vi "DimostratoreCalibrazioni.vi"() -> ()   [LabVIEW 2019]
uses:
  TypeDef/SlugExpiration.ctl
  ByteGSAPIBase.lvclass
  TypeDef/CalibrationStates.ctl
  FetchCalibration/Converted_Slug_Cluster.ctl
  Instruments/Instruments.ctl
  CalibrationMeasurements/BodyCalibrazioneMisure.ctl
  aa47c742-c095-4670-bf1f-6b28e4309cef.vi
  <vilib>/numeric/Random Number (Range) I64.vi
  <vilib>/Array/Sort 2D Array - Pop Stack.vi
  <vilib>/Array/Sort 2D Array - Push Stack.vi
  <vilib>/numeric/sub_Random U32.vi
panel:
  out "Stato":string
  out "Misurazione n.":string
  in  "Cancel":bool
  in  "Approvation":bool
  out "Tot Misurazioni":i32
  in  "Avanti":bool
  in  "Repeat":bool
  out "Esito":string
  out "Valore misurato":dbl
  out "Valore di riferimento":dbl
  out "Waveform Chart":i64(graph)
  in  "Start Calibration":bool
  in  "Next":bool
  in  "Previus":bool
  out "Calibrazioni n.":string
  in  "Filtro":enum16{"All", "Expired", "Not Expired"}(ring)
  in  "Slug list":T1[](array[typedef])
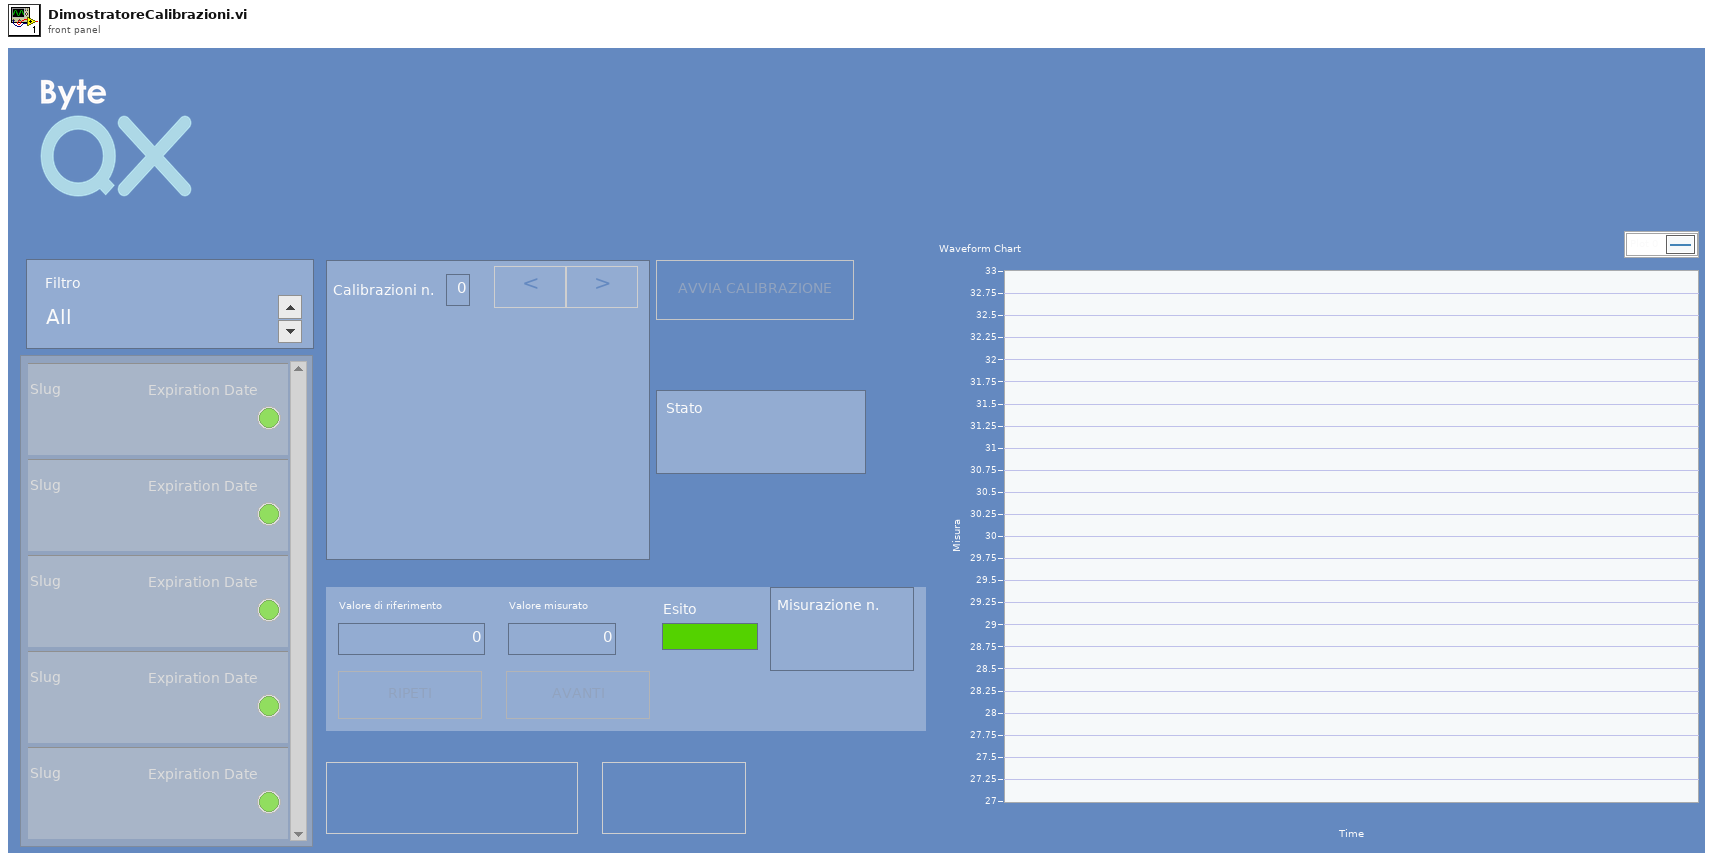
[diagram p1: front panel]
types:
  T1 = typedef "SlugExpiration.ctl" = cluster{"Slug":string, "Expiration Date":string, "Color Box":u32, "Active":bool, "Expired?":bool, "Id":i32}
  T2 = typedef "CalibrationStates.ctl" = enum16{"Init", "Idle", "GetInstruments", "Fetch", "GetCalibrations", "CheckTotalMisurations", "StartCalibration", "ManageCalibration", "AllowApprove", "Approve"}
  T3 = typedef "ByteGSWebAPI.lvlib/ByteGSAPIBase.lvclass/BodyCalibrazioneMisure.ctl" = cluster{"controls":cluster{"id":u16, "descrizione":string, "numero_misure_necessarie":u16, "riferimento_obiettivo":dbl, "mpe_max":dbl, "mpe_min":dbl, "deviazione_standard":dbl, "incertezza":dbl, "numero_misure_effettuate":u32, "temperatura_c":dbl, "umidita":dbl, "strumento_riferimento":cluster{"id":u16, "nome":string}[]}[]}
  T4 = typedef "Instruments.ctl" = cluster{"id":i32, "slug":string, "stabilimento":cluster{"id":dbl}, "categoria":cluster{"id":dbl}, "tipologia_di_visualizzazione":cluster{"id":dbl}, "stato":cluster{"id":dbl}, "descrizione":string, "costruttore":string, "matricola":string, "data_registrazione":string, "intervallo_di_taratura_mesi":dbl, "reparto":string, "campo_misura":string, "risoluzione":dbl, "responsabile_strumento":string, "classe_di_precisione":string, "classificazione":string, "appunti":string, "manuale":string, "foto":string, "riferimento":bool, "qr_hashcode":string, "costo_euro":dbl}
  T5 = typedef "ByteGSWebAPI.lvlib/ByteGSAPIBase.lvclass/Converted_Slug_Cluster.ctl" = cluster{"id":u32, "instrument":string, "name":string, "date":timestamp}
  T6 = cluster{"Esito":refnum<vi>, "Avanti":refnum<vi>, "Repeat":refnum<vi>, "Slug list":refnum<vi>, "Start Calibration":refnum<vi>, "Avanti":refnum<vi>, "Cancel":refnum<vi>, "Approvation":refnum<vi>}
  T7 = cluster{"ByteGSAPIBase in":refnum<class "ByteGSAPIBase.lvclass">, "Instruments_Slug":string[], "All_Instruments_Cals":T5[], "All_Instruments":T4[], "Slug list All":T1[], "Calibrations":T3, "Selected Slug":i32, "Misurazioni":string, "Misurazioni index":i32, "Next State":T2, "Waveform Chart":refnum<vi>, "New Val":dbl, "Id Failed":u32, "Failed?":bool, "Cal Index":i32, "Misurazioni n":string, "Stato":string, "Esito":string, "Misure effettuate":i32}
  T8 = cluster{"id":u16, "descrizione":string, "numero_misure_necessarie":u16, "riferimento_obiettivo":dbl, "mpe_max":dbl, "mpe_min":dbl, "deviazione_standard":dbl, "incertezza":dbl, "numero_misure_effettuate":u32, "temperatura_c":dbl, "umidita":dbl, "strumento_riferimento":cluster{"id":u16, "nome":string}[]}[]
  T9 = cluster{"id":u16, "descrizione":string, "numero_misure_necessarie":u16, "riferimento_obiettivo":dbl, "mpe_max":dbl, "mpe_min":dbl, "deviazione_standard":dbl, "incertezza":dbl, "numero_misure_effettuate":u32, "temperatura_c":dbl, "umidita":dbl, "strumento_riferimento":cluster{"id":u16, "nome":string}[]}
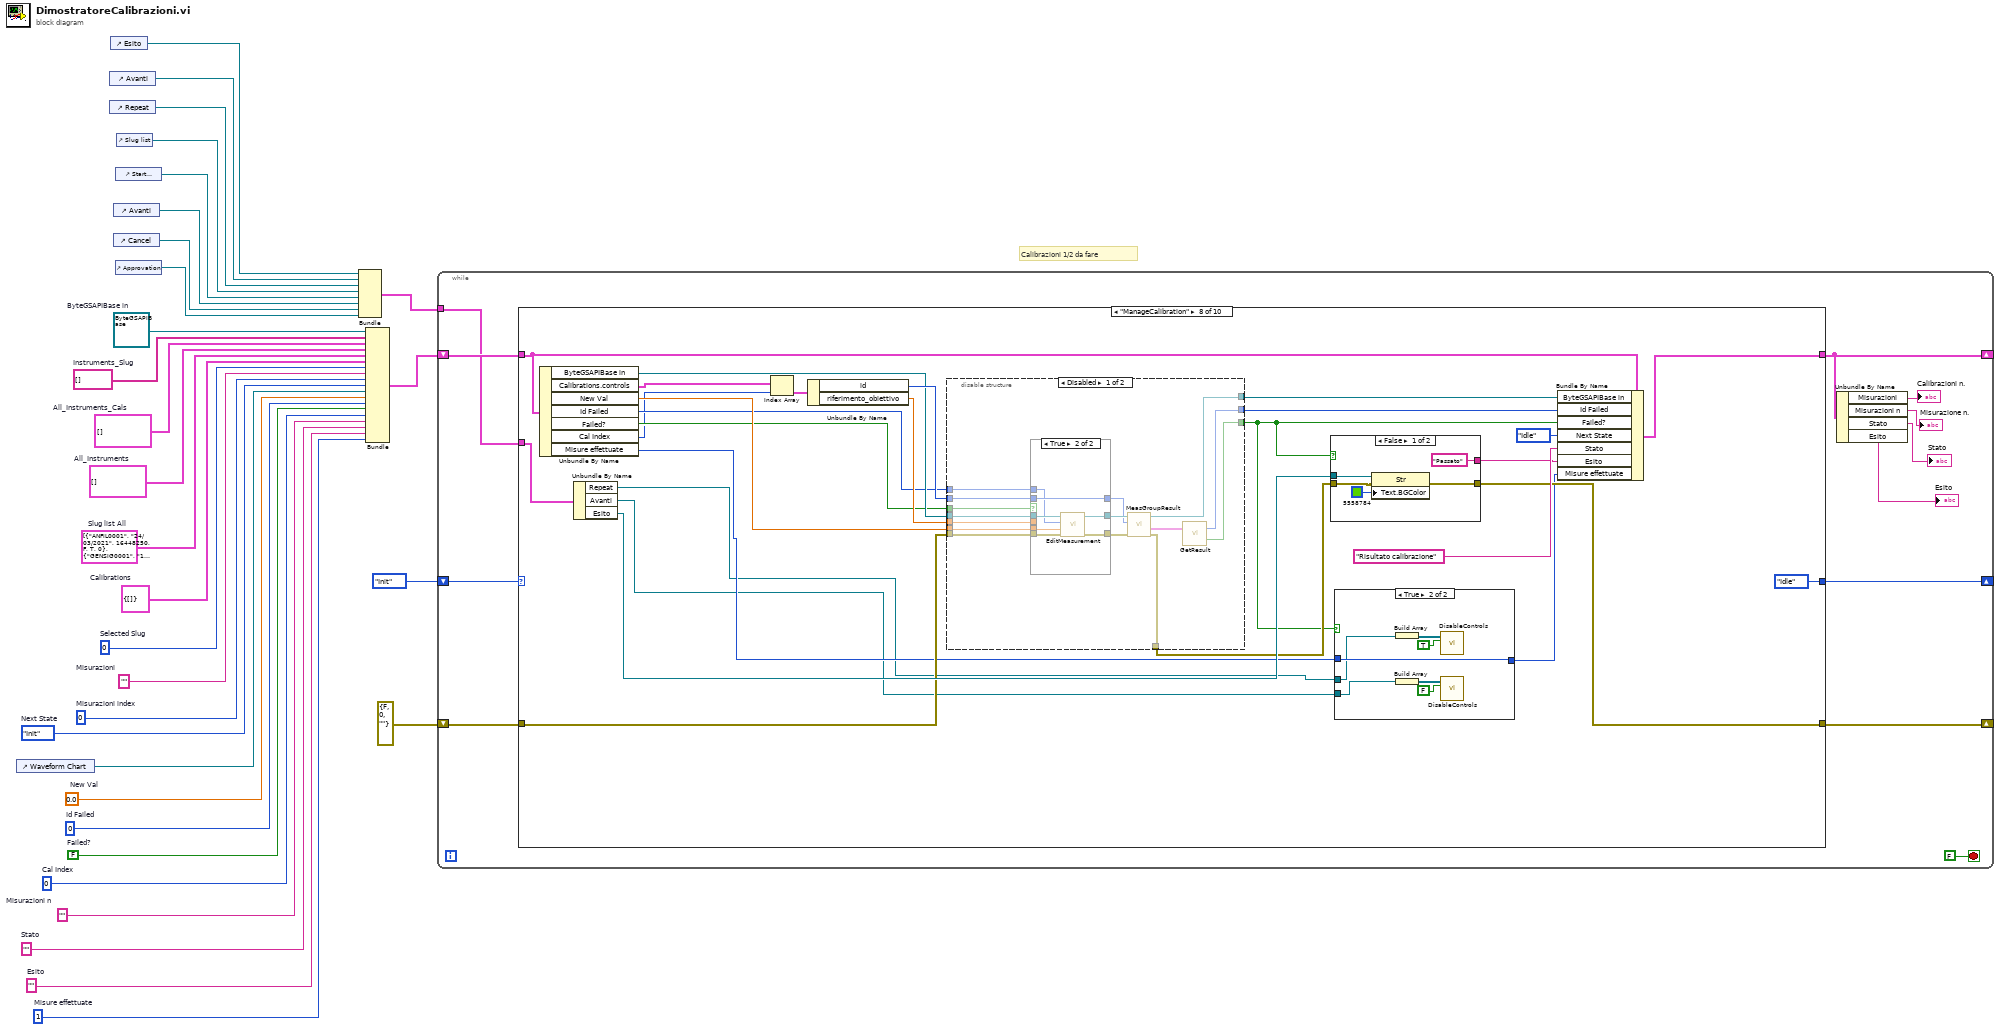
[diagram p0: block diagram]
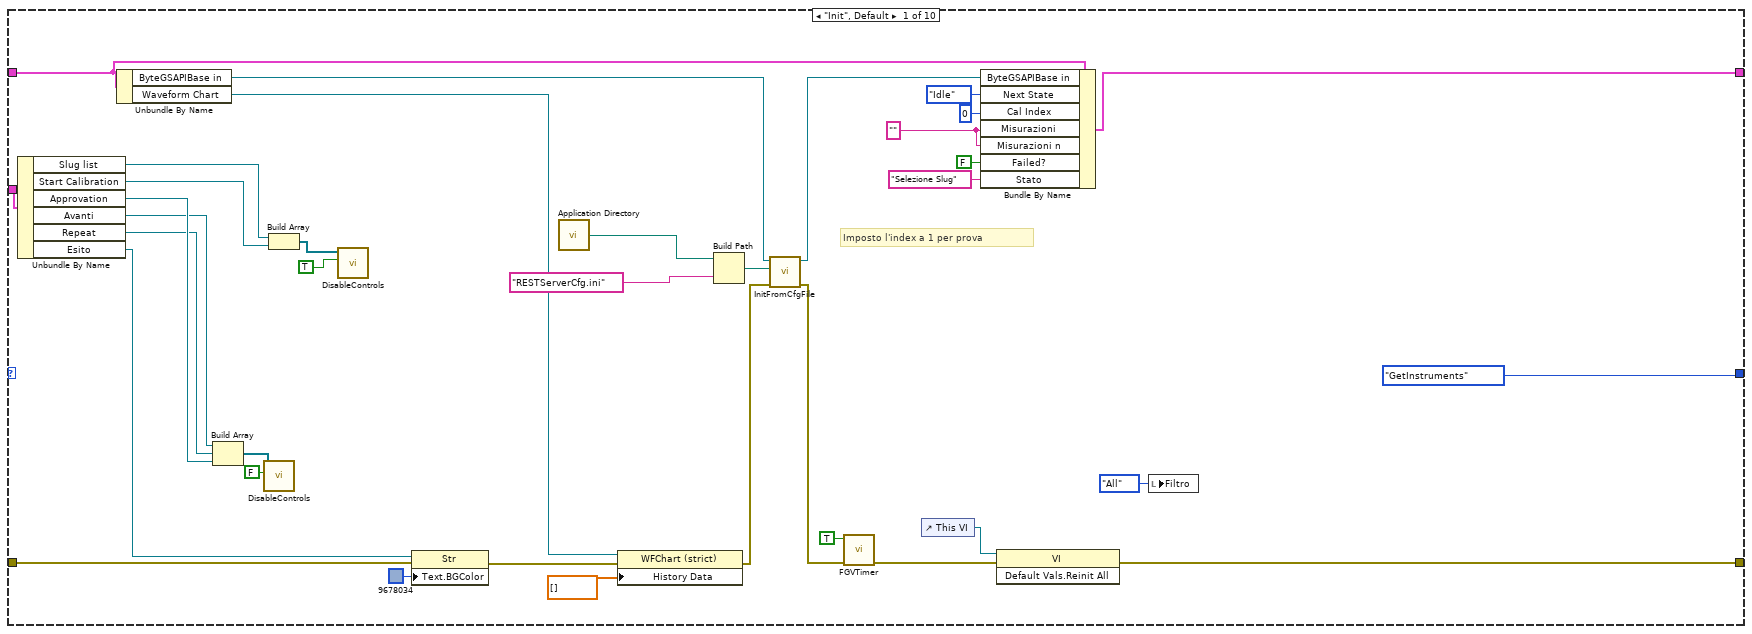
[diagram p2: hidden frame]
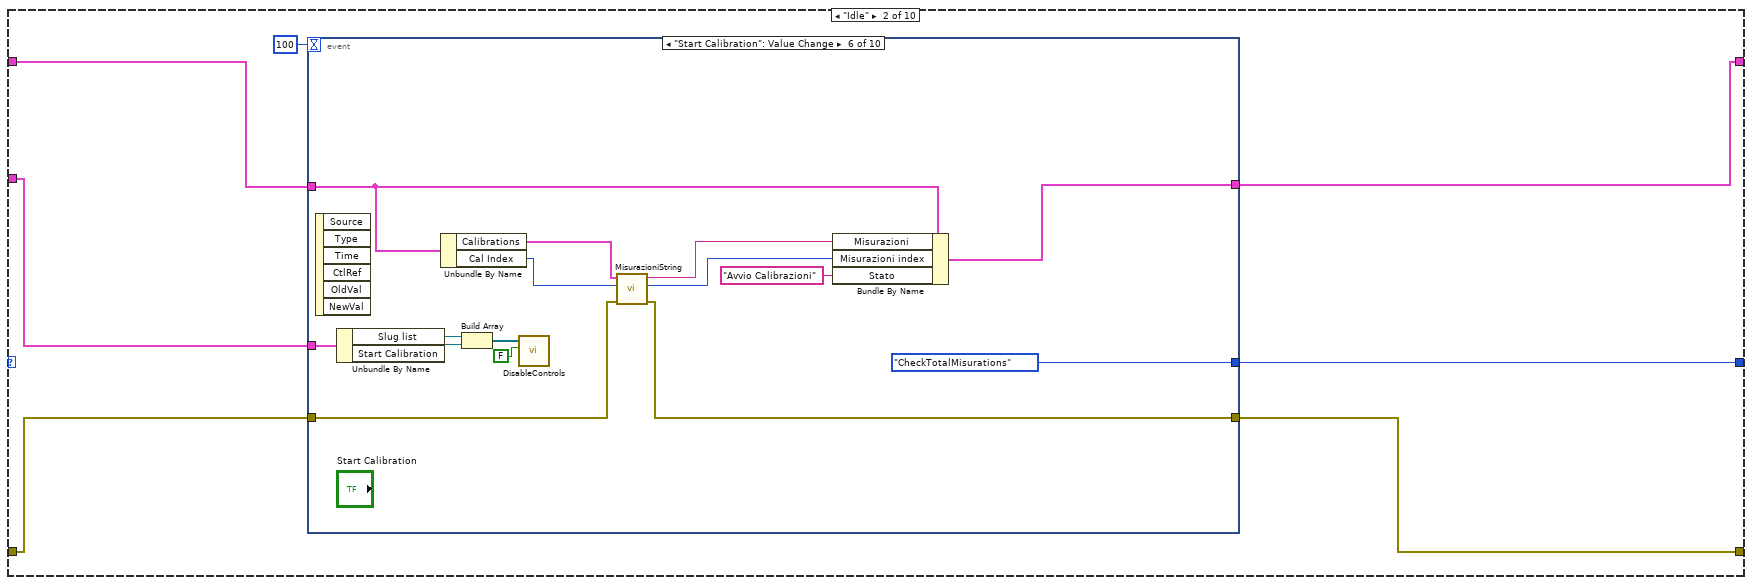
[diagram p3: hidden frame]
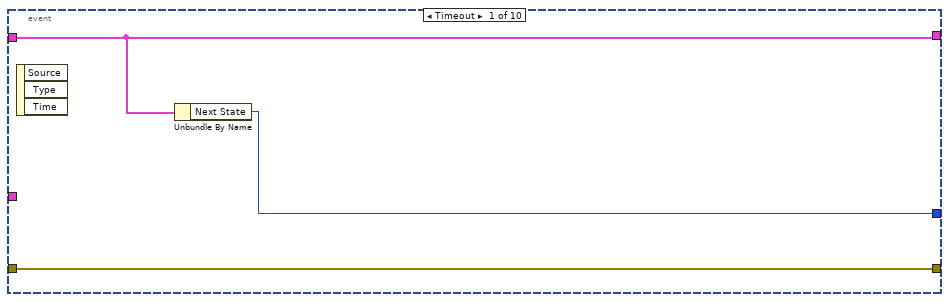
[diagram p4: hidden frame]
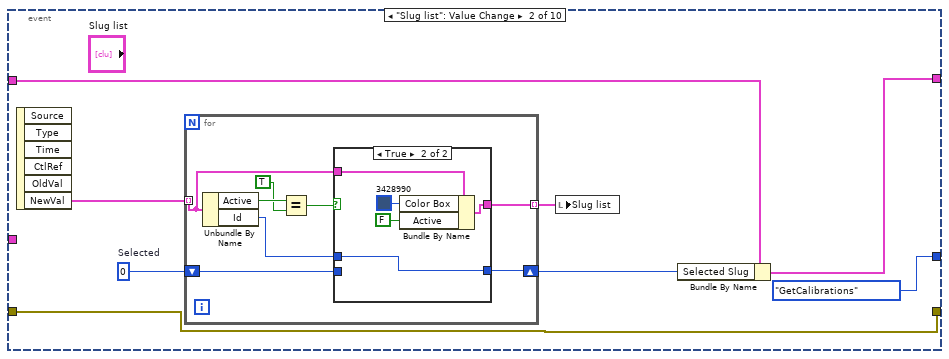
[diagram p5: hidden frame]
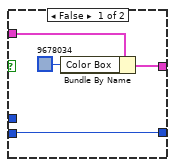
[diagram p6: hidden frame]
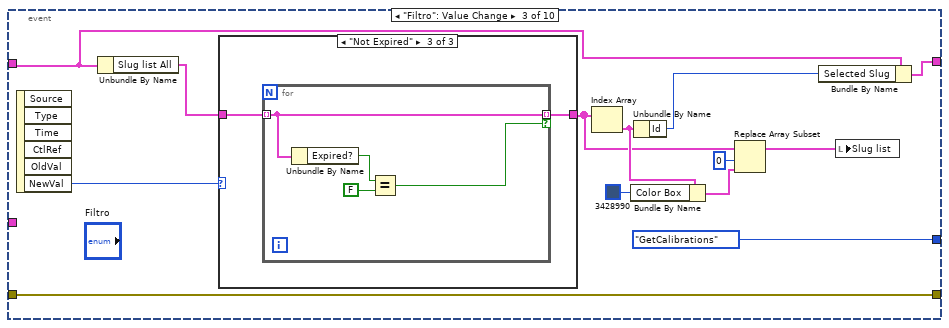
[diagram p7: hidden frame]
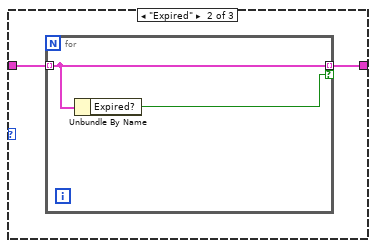
[diagram p9: hidden frame]
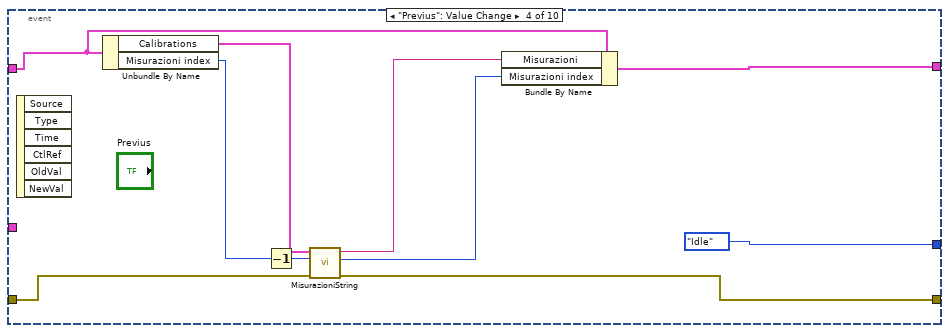
[diagram p10: hidden frame]
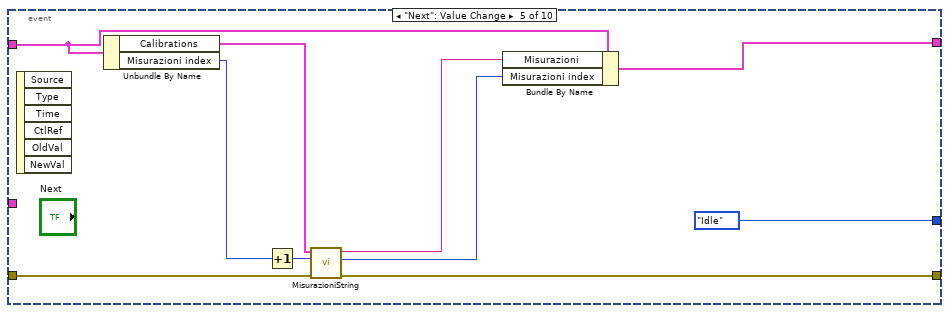
[diagram p11: hidden frame]
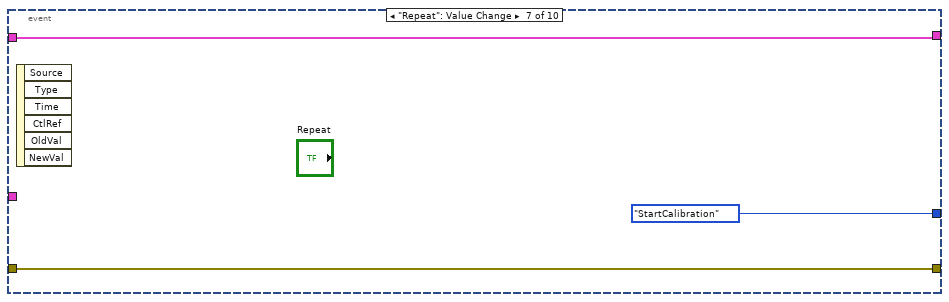
[diagram p12: hidden frame]
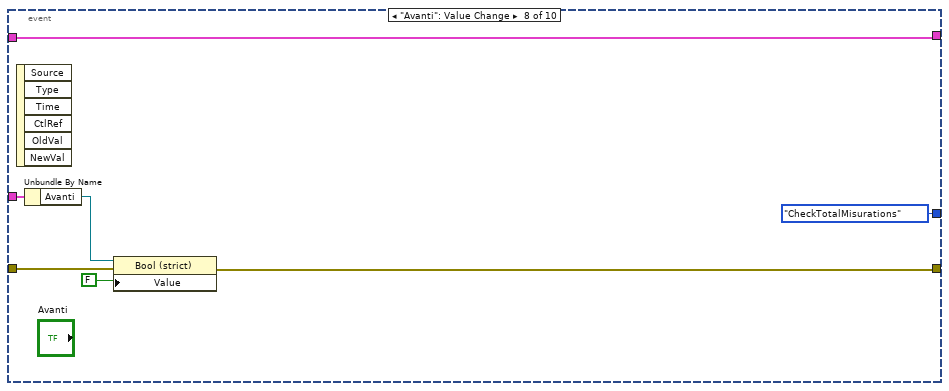
[diagram p13: hidden frame]
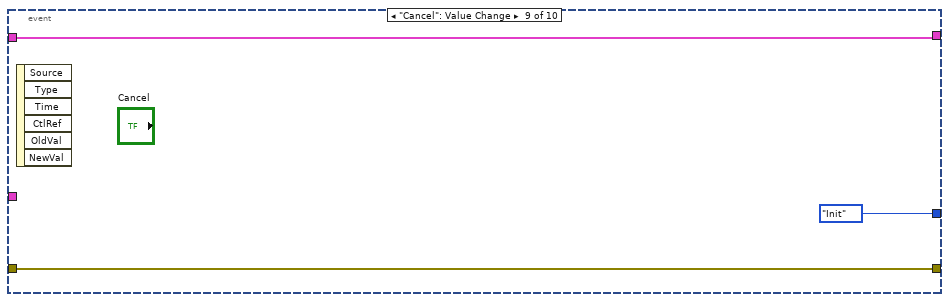
[diagram p14: hidden frame]
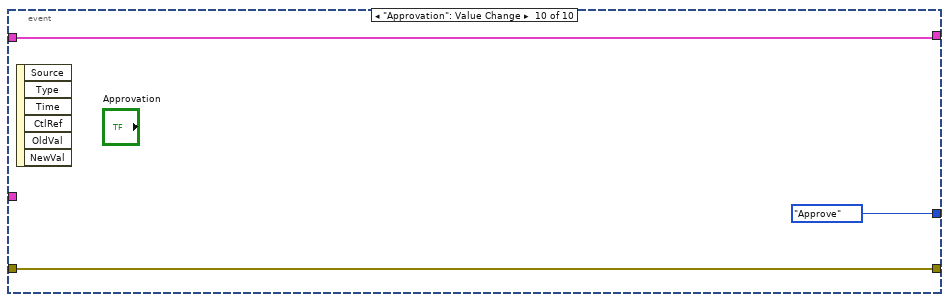
[diagram p15: hidden frame]
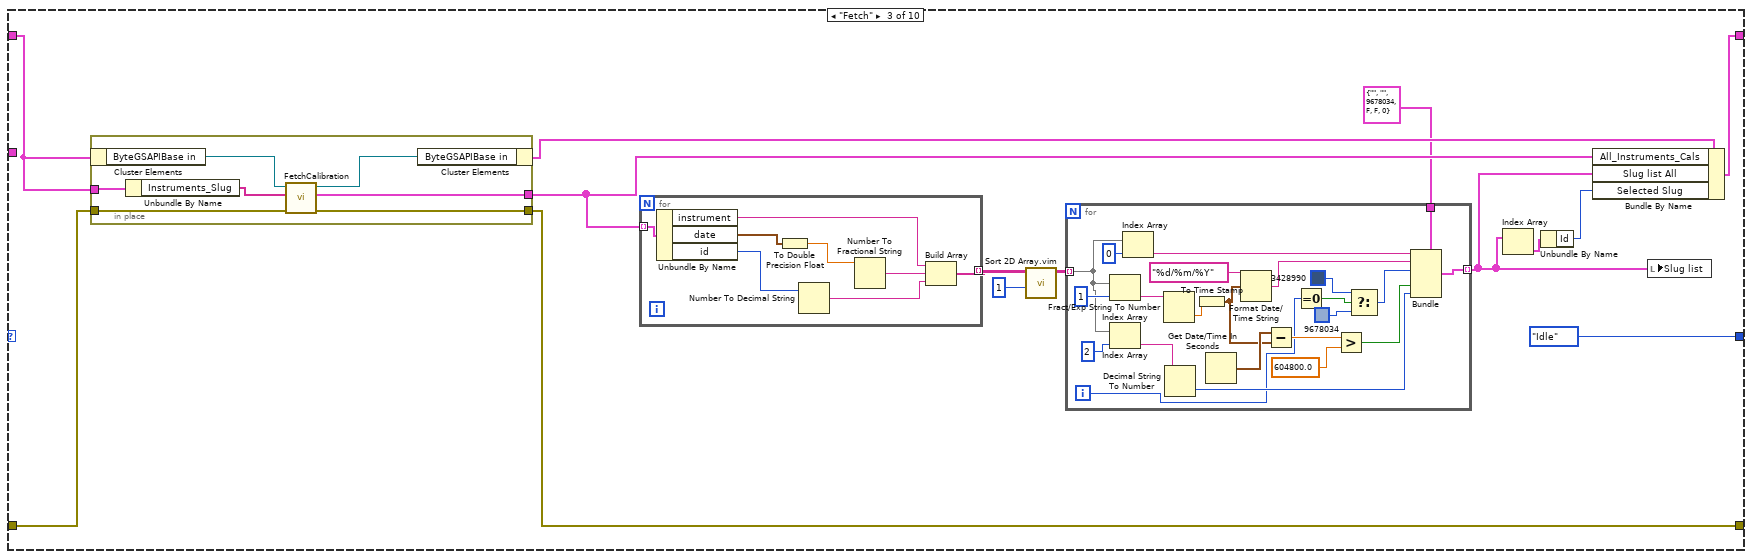
[diagram p16: hidden frame]
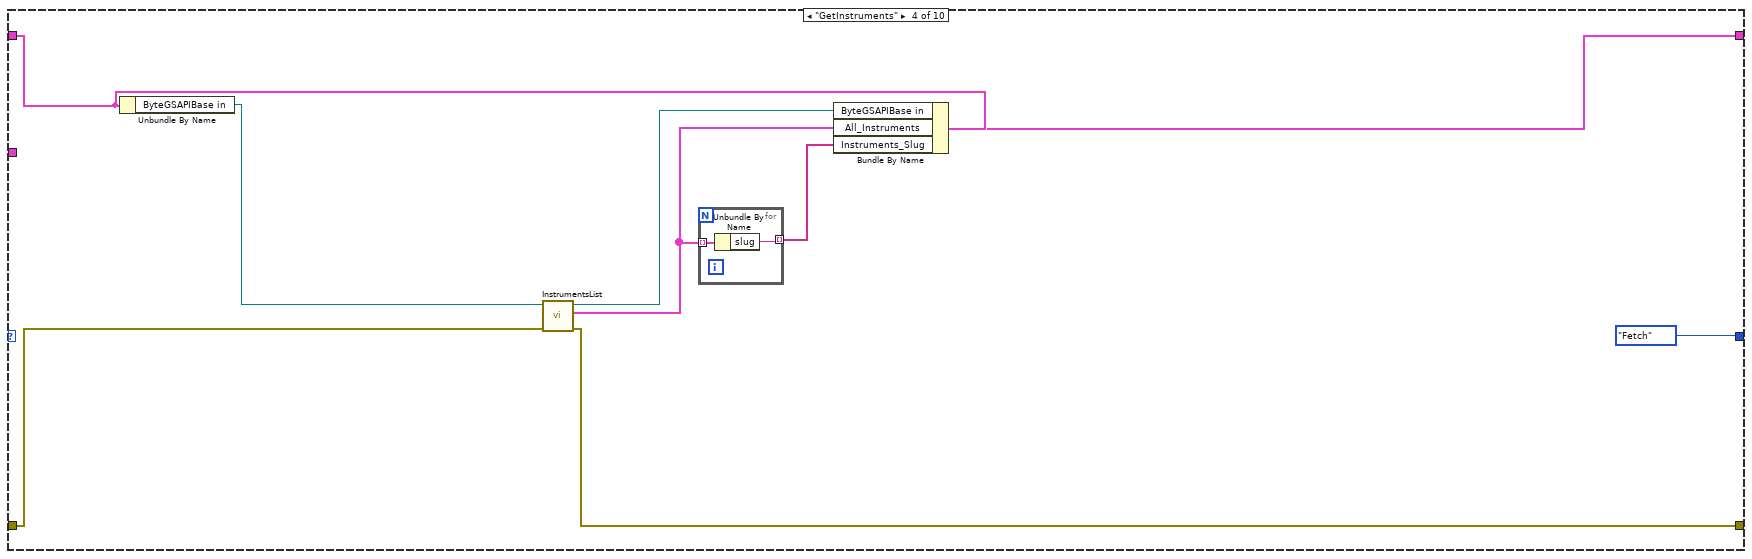
[diagram p17: hidden frame]
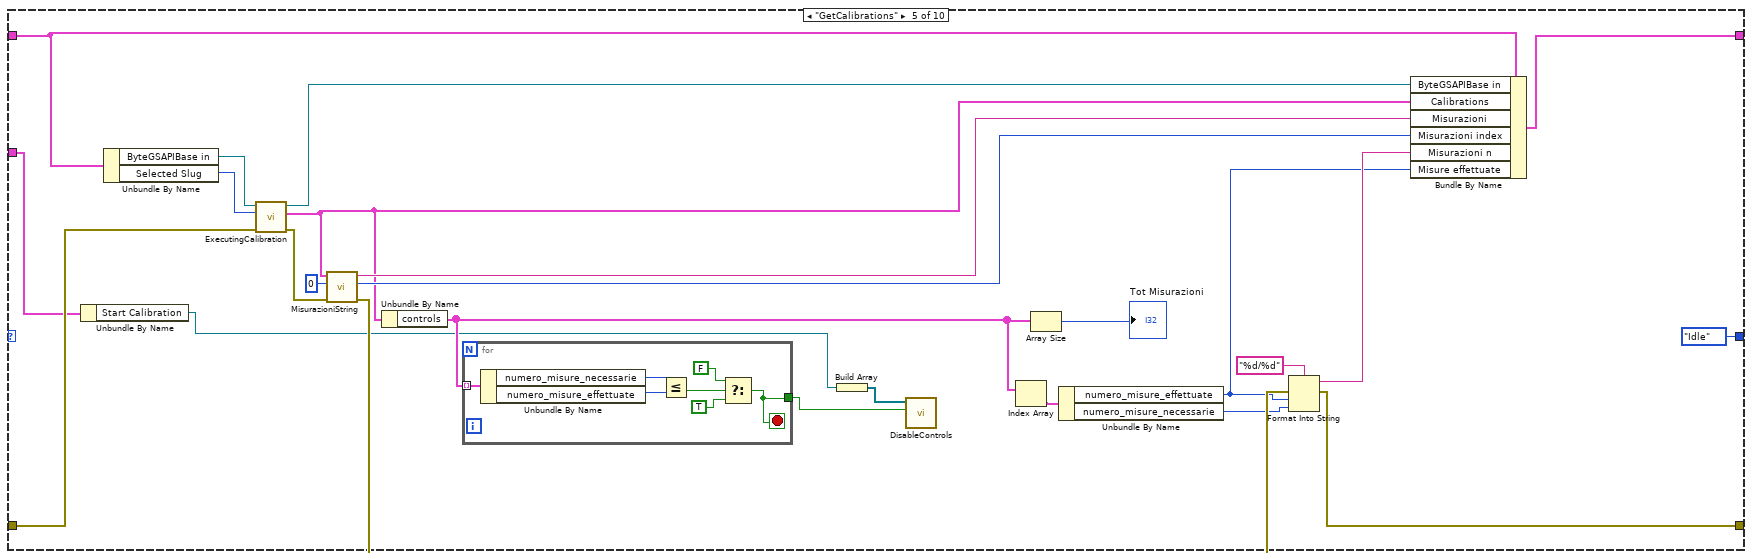
[diagram p18: hidden frame]
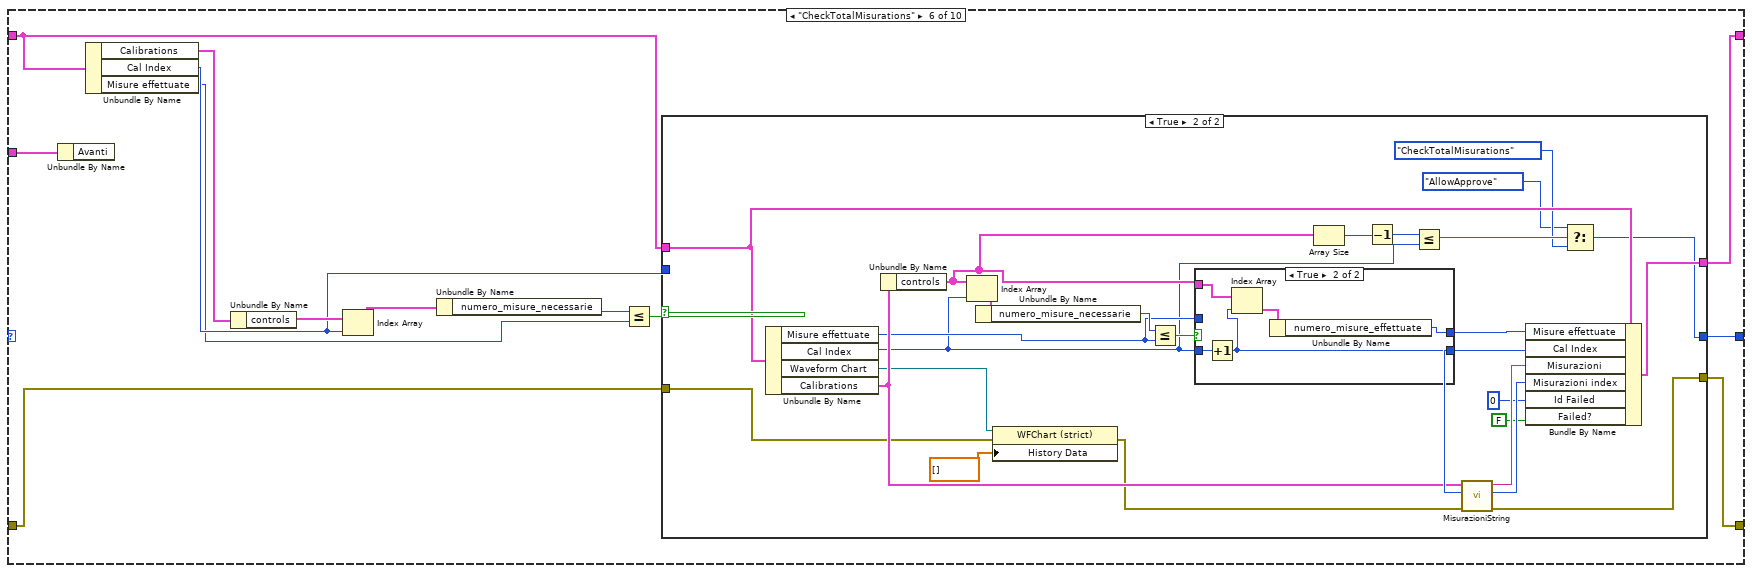
[diagram p19: hidden frame]
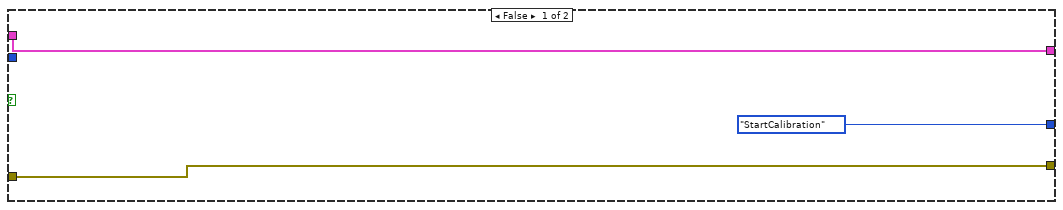
[diagram p20: hidden frame]
diagram:
  w1 = 1  # Misure effettuate
  w3 = ""  # Esito
  w4 = ""  # Stato
  w9 = ""  # Misurazioni n
  w14 = 0  # Cal Index
  w15 = FALSE  # Failed?
  w16 = u32 0  # Id Failed
  w17 = 0.0  # New Val
  w19 = CalibrationStates."Init"  # Next State
  w20 = 0  # Misurazioni index
  w21 = ""  # Misurazioni
  w22 = T1[] [{"Slug"="ANFIL0001", "Expiration Date"="24/03/2021", "Color Box"=16448250, "Active"=FALSE, "Expired?"=TRUE, "Id"=0}, {"Slug"="GENSIG0001", "Expiration Date"="18/05/2021", "Color Box"=16448250, "Active"=FALSE, "Expired?"=TRUE, "Id"=0}, {"Slug"="GENSIG0001", "Expiration Date"="15/09/2021", "Color Box"=16448250, "Active"=FALSE, "Expired?"=TRUE, "Id"=0}, {"Slug"="DIN0001", "Expiration Date"="11/10/2021", "Color Box"=13816530, "Active"=FALSE, "Expired?"=TRUE, "Id"=0}, {"Slug"="DMM0002", "Expiration Date"="20/10/2021", "Color Box"=16448250, "Active"=FALSE, "Expired?"=TRUE, "Id"=0}, {"Slug"="COMP0001", "Expiration Date"="01/12/2021", "Color Box"=16448250, "Active"=FALSE, "Expired?"=TRUE, "Id"=0}, {"Slug"="TORS0002", "Expiration Date"="06/12/2021", "Color Box"=16448250, "Active"=FALSE, "Expired?"=TRUE, "Id"=0}, {"Slug"="CDIND0001", "Expiration Date"="04/03/2022", "Color Box"=16448250, "Active"=FALSE, "Expired?"=TRUE, "Id"=0}, {"Slug"="CALI0004", "Expiration Date"="11/03/2022", "Color Box"=16448250, "Active"=FALSE, "Expired?"=TRUE, "Id"=0}, {"Slug"="CALI0001", "Expiration Date"="10/05/2022", "Color Box"=16448250, "Active"=FALSE, "Expired?"=TRUE, "Id"=0}, {"Slug"="CALI0012", "Expiration Date"="10/05/2022", "Color Box"=16448250, "Active"=FALSE, "Expired?"=TRUE, "Id"=0}, {"Slug"="CALI0011", "Expiration Date"="11/05/2022", "Color Box"=16448250, "Active"=FALSE, "Expired?"=TRUE, "Id"=0}, {"Slug"="CALI0014", "Expiration Date"="04/07/2022", "Color Box"=16448250, "Active"=FALSE, "Expired?"=TRUE, "Id"=0}, {"Slug"="CDIND0001", "Expiration Date"="15/07/2022", "Color Box"=16448250, "Active"=FALSE, "Expired?"=TRUE, "Id"=0}, {"Slug"="CALI0024", "Expiration Date"="11/07/2023", "Color Box"=16448250, "Active"=FALSE, "Expired?"=TRUE, "Id"=0}, {"Slug"="CALI0017", "Expiration Date"="19/09/2023", "Color Box"=16448250, "Active"=FALSE, "Expired?"=TRUE, "Id"=0}, {"Slug"="CALI0020", "Expiration Date"="02/11/2023", "Color Box"=16448250, "Active"=FALSE, "Expired?"=TRUE, "Id"=0}, {"Slug"="CALI0017", "Expiration Date"="03/11/2023", "Color Box"=16448250, "Active"=FALSE, "Expired?"=TRUE, "Id"=0}, {"Slug"="CALI0025", "Expiration Date"="11/11/2023", "Color Box"=16448250, "Active"=FALSE, "Expired?"=TRUE, "Id"=0}, {"Slug"="CLBR0001", "Expiration Date"="30/11/2023", "Color Box"=16448250, "Active"=FALSE, "Expired?"=TRUE, "Id"=0}, {"Slug"="CLBR0001", "Expiration Date"="02/01/2024", "Color Box"=16448250, "Active"=FALSE, "Expired?"=TRUE, "Id"=0}, {"Slug"="CLBR0001", "Expiration Date"="02/01/2024", "Color Box"=16448250, "Active"=FALSE, "Expired?"=TRUE, "Id"=0}, {"Slug"="CLBR0003", "Expiration Date"="04/03/2024", "Color Box"=16448250, "Active"=FALSE, "Expired?"=TRUE, "Id"=0}, {"Slug"="MICP0001", "Expiration Date"="19/03/2024", "Color Box"=16448250, "Active"=FALSE, "Expired?"=TRUE, "Id"=0}, {"Slug"="TERM0002", "Expiration Date"="04/07/2024", "Color Box"=16448250, "Active"=FALSE, "Expired?"=TRUE, "Id"=0}, {"Slug"="ACCEL0008", "Expiration Date"="04/07/2024", "Color Box"=16448250, "Active"=FALSE, "Expired?"=TRUE, "Id"=0}, {"Slug"="ACCEL0008", "Expiration Date"="05/07/2024", "Color Box"=16448250, "Active"=FALSE, "Expired?"=TRUE, "Id"=0}, {"Slug"="ACCEL0008", "Expiration Date"="19/08/2024", "Color Box"=16448250, "Active"=FALSE, "Expired?"=TRUE, "Id"=0}, {"Slug"="TERM0002", "Expiration Date"="15/10/2024", "Color Box"=16448250, "Active"=FALSE, "Expired?"=TRUE, "Id"=0}, {"Slug"="BILA0001", "Expiration Date"="15/10/2024", "Color Box"=16448250, "Active"=FALSE, "Expired?"=TRUE, "Id"=0}, {"Slug"="CLBR0001", "Expiration Date"="15/10/2024", "Color Box"=16448250, "Active"=FALSE, "Expired?"=TRUE, "Id"=0}, {"Slug"="ACCEL0002", "Expiration Date"="15/10/2024", "Color Box"=16448250, "Active"=FALSE, "Expired?"=TRUE, "Id"=0}]  # Slug list All
  w23 = 0  # Selected Slug
  w24 = T3 {"controls"=[]}  # Calibrations
  w25 = T4[] []  # All_Instruments
  w26 = T5[] []  # All_Instruments_Cals
  w27 = string[] []  # Instruments_Slug
  w30 = refnum<class "ByteGSAPIBase.lvclass"> refnum  # ByteGSAPIBase in
  # "Calibrazioni 1/2 da fare"
  n1 = control-ref of="Waveform Chart"() -> (w18:refnum<vi>)
  n2 = control-ref of="Avanti"() -> (w5:refnum<vi>)
  n3 = control-ref of="Repeat"() -> (w6:refnum<vi>)
  n4 = control-ref of="Esito"() -> (w2:refnum<vi>)
  n5 = control-ref of="Avanti"() -> (w10:refnum<vi>)
  n6 = control-ref of="Cancel"() -> (w11:refnum<vi>)
  n7 = control-ref of="Start Calibration"() -> (w8:refnum<vi>)
  n8 = control-ref of="Approvation"() -> (w12:refnum<vi>)
  n9 = control-ref of="Slug list"() -> (w7:refnum<vi>)
  n10 = Bundle("Esito"=w2, "Avanti"=w5, "Repeat"=w6, "Slug list"=w7, "Start Calibration"=w8, "Avanti"=w10, "Cancel"=w11, "Approvation"=w12) -> (w13:T6)  [unwired: 1 in]
  n11 = Bundle("ByteGSAPIBase in"=w30, "Instruments_Slug"=w27, "All_Instruments_Cals"=w26, "All_Instruments"=w25, "Slug list All"=w22, "Calibrations"=w24, "Selected Slug"=w23, "Misurazioni"=w21, "Misurazioni index"=w20, "Next State"=w19, "Waveform Chart"=w18, "New Val"=w17, "Id Failed"=w16, "Failed?"=w15, "Cal Index"=w14, "Misurazioni n"=w9, "Stato"=w4, "Esito"=w3, "Misure effettuate"=w1) -> (w29:T7)  [unwired: 1 in]
  n12 = while {
    shift-right: [w41] -> _
    shift-left: CalibrationStates."Init" -> [w42]
    shift-right: [w37] -> _
    shift-left: w29 -> [w40]
    shift-right: [w38] -> _
    shift-left: errorcluster {"status"=FALSE, "code"=0, "source"=""} ("error in (no error)") -> [w39]
    tunnel: w13 -> [w35]
    stop <- FALSE stop-if-true
    n13 = case shown="\"ManageCalibration\"" w42 {
      tunnel: [CalibrationStates."GetInstruments" w84 CalibrationStates."Idle" CalibrationStates."Fetch" CalibrationStates."Idle" w292 CalibrationStates."Idle" CalibrationStates."Idle" CalibrationStates."Idle" CalibrationStates."Idle"] -> w41
      tunnel: w40 -> [w75 w86 w203 w248 w273 w288 w359 w395 w462 w496]
      tunnel: w39 -> [w45 w83 w202 w250 w274 w290 w343 w381 w465 w495]
      tunnel: [w61 w82 w195 w244 w264 w289 w351 w382 w465 w493] -> w38
      tunnel: [w73 w85 w199 w246 w272 w287 w358 w394 w462 w487] -> w37
      tunnel: w35 -> [w63 w80 _ _ w256 w291 w347 w387 w471 w492]
      frame "Init", Default {
        w59 = "" ("Misurazioni")
        # "Imposto l'index a 1 per prova"
        n14 = Unbundle By Name(w63) -> ("Slug list"=w57:refnum<vi>, "Start Calibration"=w56:refnum<vi>, "Approvation"=w58:refnum<vi>, "Avanti"=w51:refnum<vi>, "Repeat"=w50:refnum<vi>, "Esito"=w44:refnum<vi>)
        n15 = Unbundle By Name(w75) -> ("ByteGSAPIBase in"=w76:refnum<class "ByteGSAPIBase.lvclass">, "Waveform Chart"=w67:refnum<vi>)
        n16 = Build Array(w51, w50, w58) -> (w53:refnum<vi>[])
        n17 = call "DisableControls.vi"("Visible"=FALSE, "Controls"=w53) -> ()  [unwired: 9 in, 1 out]
        n18 = Build Array(w57, w56) -> (w55:refnum<vi>[])
        n19 = call "DisableControls.vi"("Visible"=TRUE, "Controls"=w55) -> ()  [unwired: 9 in, 1 out]
        n20 = property class="Str"(reference=w44, error in=w45, "Text.BGColor"=u32 9678034 ("Text.Text Colors:BG Color")) -> (error out=w46:errorcluster)  [unwired: 1 out]
        n21 = call <vilib>:"Application Directory.vi"() -> ("Application Directory"=w77:path)
        n22 = property class="WFChart (strict)"(reference=w67, error in=w46, "History Data"=dbl[] []) -> (error out=w66:errorcluster)  [unwired: 1 out]
        n23 = Build Path(base path=w77, name or relative path="RESTServerCfg.ini") -> (appended path=w72:path)
        n24 = call-dynamic "InitFromCfgFile.vi"("error in (no error)"=w66, "configuration file path"=w72, "ByteGSAPIBase in"=w76) -> ("error out"=w70:errorcluster, "ByteGSAPIBase out"=w74:refnum<class "ByteGSAPIBase.lvclass">)  [unwired: 7 in]
        n25 = call "FGVTimer.vi"("error in"=w70, "Reset"=TRUE) -> ("error out"=w62:errorcluster)  [unwired: 7 in, 2 out]
        n26 = control-ref of="This VI"() -> (w60:refnum<vi>)
        n27 = Bundle By Name(cluster=w75, "ByteGSAPIBase in"=w74, "Next State"=CalibrationStates."Idle", "Cal Index"=0, "Misurazioni"=w59, "Misurazioni n"=w59, "Failed?"=FALSE, "Stato"="Selezione Slug") -> (w73:T7)
        n28 = invoke class="VI" method="Default Vals.Reinit All"(reference=w60, error in=w62) -> (error out=w61:errorcluster)  [unwired: 1 in, 2 out]
        n29 = local write "Filtro"(enum16{"All", "Expired", "Not Expired"}."All" ("Filter")) -> ()
      }
      frame "Idle" {
        n30 = event shown="[5] \"Start Calibration\": Value Change" {
          selector: _ -> [_ _ _ _ _ _ _ _ _ _]
          dyn-events: _ -> [_ _ _ _ _ _ _ _ _ _]
          timeout: 100 -> [_ _ _ _ _ _ _ _ _ _]
          tunnel: w86 -> [w88 w94 w123 w143 w153 w170 w176 w177 w184 w187]
          tunnel: [w88 w92 w122 w142 w150 w167 w176 w177 w184 w187] -> w85
          tunnel: [w87 CalibrationStates."GetCalibrations" CalibrationStates."GetCalibrations" CalibrationStates."Idle" CalibrationStates."Idle" CalibrationStates."CheckTotalMisurations" CalibrationStates."StartCalibration" CalibrationStates."CheckTotalMisurations" CalibrationStates."Init" CalibrationStates."Approve"] -> w84
          tunnel: w83 -> [w89 w90 w124 w140 w158 w166 w174 w178 w186 w189]
          tunnel: [w89 w90 w124 w139 w157 w164 w174 w179 w186 w189] -> w82
          tunnel: w80 -> [_ _ _ _ _ w165 _ w180 _ _]
          event Timeout {
            n31 = event-data() -> ()  [unwired: 1 in, 3 out]
            n32 = Unbundle By Name(w88) -> ("Next State"=w87:T2)
          }
          event "Slug list": Value Change {
            w95 = 0  # Selected
            n33 = event-data() -> ("NewVal"=w97:T1[])  [unwired: 1 in, 5 out]
            n34 = for {
              tunnel: w97 -> [w102] mode=indexing
              tunnel: [w101] -> w96 mode=indexing
              shift-right: [w99] -> w93
              shift-left: w95 -> [w100]
              n35 = Unbundle By Name(w102) -> ("Active"=w105:bool, "Id"=w98:i32)
              n36 = Equal?(x=w105, y=TRUE) -> (x = y?=w103:bool)
              n37 = case shown="True" w103 {
                tunnel: w102 -> [w108 w114]
                tunnel: [w109 w112] -> w101
                tunnel: w100 -> [w106 _]
                tunnel: [w106 w110] -> w99
                tunnel: w98 -> [_ w110]
                frame False {
                  n38 = Bundle By Name(cluster=w108, "Color Box"=u32 9678034) -> (w109:T1)
                }
                frame True {
                  n39 = Bundle By Name(cluster=w114, "Color Box"=u32 3428990, "Active"=FALSE) -> (w112:T1)
                }
              }
            }
            n40 = local write "Slug list"(w96) -> ()
            n41 = Bundle By Name(cluster=w94, "Selected Slug"=w93) -> (w92:T7)
          }
          event "Filtro": Value Change {
            n42 = event-data() -> ("NewVal"=w127:enum16{"All", "Expired", "Not Expired"})  [unwired: 1 in, 5 out]
            n43 = Unbundle By Name(w123) -> ("Slug list All"=w126:T1[])
            n44 = case shown="\"Not Expired\"" w127 {
              tunnel: w126 -> [w128 w130 w134]
              tunnel: [w128 w129 w133] -> w118
              frame "All" {
              }
              frame "Expired" {
                n45 = for {
                  tunnel: w130 -> [w132] mode=indexing
                  tunnel: [w132] -> w129 mode=indexing if=w131
                  n46 = Unbundle By Name(w132) -> ("Expired?"=w131:bool)
                }
              }
              frame "Not Expired" {
                n47 = for {
                  tunnel: w134 -> [w138] mode=indexing
                  tunnel: [w138] -> w133 mode=indexing if=w135
                  n48 = Unbundle By Name(w138) -> ("Expired?"=w137:bool)
                  n49 = Equal?(x=w137, y=FALSE) -> (x = y?=w135:bool)
                }
              }
            }
            n50 = Index Array(array=w118) -> (element=w120:T1)  [unwired: 1 in]
            n51 = Bundle By Name(cluster=w120, "Color Box"=u32 3428990) -> (w117:T1)
            n52 = Unbundle By Name(w120) -> ("Id"=w121:i32)
            n53 = Replace Array Subset(array=w118, new element=w117, index=0) -> (w115:T1[])
            n54 = Bundle By Name(cluster=w123, "Selected Slug"=w121) -> (w122:T7)
            n55 = local write "Slug list"(w115) -> ()
          }
          event "Previus": Value Change {
            n56 = event-data() -> ()  [unwired: 1 in, 6 out]
            n57 = Unbundle By Name(w143) -> ("Calibrations"=w148:T3, "Misurazioni index"=w146:i32)
            n58 = Decrement(x=w146) -> (x-1=w147:i32)
            n59 = call "MisurazioniString.vi"("error in (no error)"=w140, "index"=w147, "Calibration data"=w148) -> ("error out"=w139:errorcluster, "index"=w144:i32, "String"=w145:string)  [unwired: 6 in]
            n60 = Bundle By Name(cluster=w143, "Misurazioni"=w145, "Misurazioni index"=w144) -> (w142:T7)
          }
          event "Next": Value Change {
            n61 = event-data() -> ()  [unwired: 1 in, 6 out]
            n62 = Unbundle By Name(w153) -> ("Calibrations"=w156:T3, "Misurazioni index"=w154:i32)
            n63 = Increment(x=w154) -> (x+1=w155:i32)
            n64 = call "MisurazioniString.vi"("error in (no error)"=w158, "index"=w155, "Calibration data"=w156) -> ("error out"=w157:errorcluster, "index"=w151:i32, "String"=w152:string)  [unwired: 6 in]
            n65 = Bundle By Name(cluster=w153, "Misurazioni"=w152, "Misurazioni index"=w151) -> (w150:T7)
          }
          event "Start Calibration": Value Change {
            n66 = event-data() -> ()  [unwired: 1 in, 6 out]
            n67 = Unbundle By Name(w165) -> ("Slug list"=w163:refnum<vi>, "Start Calibration"=w162:refnum<vi>)
            n68 = Unbundle By Name(w170) -> ("Calibrations"=w172:T3, "Cal Index"=w171:i32)
            n69 = Build Array(w163, w162) -> (w161:refnum<vi>[])
            n70 = call "DisableControls.vi"("Visible"=FALSE, "Controls"=w161) -> ()  [unwired: 9 in, 1 out]
            n71 = call "MisurazioniString.vi"("error in (no error)"=w166, "index"=w171, "Calibration data"=w172) -> ("error out"=w164:errorcluster, "index"=w168:i32, "String"=w169:string)  [unwired: 6 in]
            n72 = Bundle By Name(cluster=w170, "Misurazioni"=w169, "Misurazioni index"=w168, "Stato"="Avvio Calibrazioni") -> (w167:T7)
          }
          event "Repeat": Value Change {
            n73 = event-data() -> ()  [unwired: 1 in, 6 out]
          }
          event "Avanti": Value Change {
            n74 = event-data() -> ()  [unwired: 1 in, 6 out]
            n75 = Unbundle By Name(w180) -> ("Avanti"=w182:refnum<vi>)
            n76 = property class="Bool (strict)"(reference=w182, error in=w178, "Value"=FALSE) -> (error out=w179:errorcluster)  [unwired: 1 out]
          }
          event "Cancel": Value Change {
            n77 = event-data() -> ()  [unwired: 1 in, 6 out]
          }
          event "Approvation": Value Change {
            n78 = event-data() -> ()  [unwired: 1 in, 6 out]
          }
        }
      }
      frame "Fetch" {
        n79 = in-place {
          in-place-border: w202 -> [w240]
          in-place-border: [w239] -> w195
          in-place-border: [w238] -> w194
          in-place-border: w203 -> [w236]
          n80 = in-place-cluster #1(w203) -> ("ByteGSAPIBase in"=w237:refnum<class "ByteGSAPIBase.lvclass">)
          n81 = Unbundle By Name(w236) -> ("Instruments_Slug"=w235:string[])
          n82 = call "FetchCalibration.vi"("error in (no error)"=w240, "Instruments"=w235, "ByteGSAPIBase in"=w237) -> ("error out"=w239:errorcluster, "Instruments"=w238:T5[], "ByteGSAPIBase out"=w241:refnum<class "ByteGSAPIBase.lvclass">)  [unwired: 6 in]
          n83 = in-place-cluster #1("ByteGSAPIBase in"=w241) -> (w200:T7)
        }
        n84 = for {
          tunnel: w194 -> [w234] mode=indexing
          tunnel: [w233] -> w198 mode=indexing
          n85 = Unbundle By Name(w234) -> ("instrument"=w232:string, "date"=w231:timestamp, "id"=w228:u32)
          n86 = To Double Precision Float(number=w231) -> (double precision float=w230:dbl)
          n87 = Number To Decimal String(number=w228) -> (decimal integer string=w227:string)  [unwired: 1 in]
          n88 = Number To Fractional String(number=w230) -> (F-format string=w229:string)  [unwired: 3 in]
          n89 = Build Array(w232, w229, w227) -> (w233:string[])
        }
        n90 = call "Sort 2D Array.vim"("index"=1, "2D array"=w198) -> ("sorted 2D array"=w196:string[][])  [unwired: 8 in, 1 out]
        n91 = for {
          tunnel: w196 -> [w211] mode=indexing
          tunnel: T1 {"Slug"="", "Expiration Date"="", "Color Box"=9678034, "Active"=FALSE, "Expired?"=FALSE, "Id"=0} ("Slug list 2") -> [w226]
          tunnel: [w218] -> w192 mode=indexing
          i -> [w208]
          n92 = Index Array(array=w211, index=1) -> (element=w222:string)
          n93 = Index Array(array=w211, index=2) -> (element=w210:string)
          n94 = Index Array(array=w211, index=0) -> (element=w224:string)
          n95 = Fract/Exp String To Number(string=w222) -> (number=w221:dbl)  [unwired: 3 in, 1 out]
          n96 = Decimal String To Number(string=w210) -> (number=w209:i32)  [unwired: 2 in, 1 out]
          n97 = To Time Stamp(1:w221) -> (0:w213:timestamp)
          n98 = Get Date/Time In Seconds() -> (seconds since 1Jan1904=w214:timestamp)
          n99 = Format Date/Time String(time format string (%c)="%d/%m/%Y", seconds (now)=w213) -> (date/time string=w219:string)  [unwired: 1 in]
          n100 = Subtract(x=w214, y=w213) -> (x-y=w217:dbl)
          n101 = Equal To 0?(x=w208) -> (x = 0?=w207:bool)
          n102 = Greater?(x=w217, y=604800.0) -> (0:w215:bool)
          n103 = Select(t=u32 3428990 ("Color Box"), s=w207, f=u32 9678034 ("Color Box")) -> (s? t:f=w204:u32)
          n104 = Bundle(cluster=w226, "Slug"=w224, "Expiration Date"=w219, "Color Box"=w204, "Expired?"=w215, "Id"=w209) -> (w218:T1)  [unwired: 1 in]
        }
        n105 = Index Array(array=w192) -> (element=w191:T1)  [unwired: 1 in]
        n106 = Unbundle By Name(w191) -> ("Id"=w190:i32)
        n107 = Bundle By Name(cluster=w200, "All_Instruments_Cals"=w194, "Slug list All"=w192, "Selected Slug"=w190) -> (w199:T7)
        n108 = local write "Slug list"(w192) -> ()
      }
      frame "GetInstruments" {
        n109 = Unbundle By Name(w248) -> ("ByteGSAPIBase in"=w249:refnum<class "ByteGSAPIBase.lvclass">)
        n110 = call "InstrumentsList.vi"("error in (no error)"=w250, "ByteGSAPIBase in"=w249) -> ("error out"=w244:errorcluster, "Array"=w243:T4[], "ByteGSAPIBase out"=w247:refnum<class "ByteGSAPIBase.lvclass">)  [unwired: 7 in]
        n111 = for {
          tunnel: w243 -> [w252] mode=indexing
          tunnel: [w251] -> w242 mode=indexing
          n112 = Unbundle By Name(w252) -> ("slug"=w251:string)
        }
        n113 = Bundle By Name(cluster=w248, "ByteGSAPIBase in"=w247, "All_Instruments"=w243, "Instruments_Slug"=w242) -> (w246:T7)
      }
      frame "GetCalibrations" {
        n114 = Unbundle By Name(w256) -> ("Start Calibration"=w255:refnum<vi>)
        n115 = Unbundle By Name(w273) -> ("ByteGSAPIBase in"=w275:refnum<class "ByteGSAPIBase.lvclass">, "Selected Slug"=w276:i32)
        n116 = call "ExecutingCalibration.vi"("error in (no error)"=w274, "calibration_id"=w276, "ByteGSAPIBase in"=w275) -> ("error out"=w270:errorcluster, "Calibration data"=w266:T3, "ByteGSAPIBase out"=w271:refnum<class "ByteGSAPIBase.lvclass">)  [unwired: 6 in]
        n117 = call "MisurazioniString.vi"("error in (no error)"=w270, "index"=0, "Calibration data"=w266) -> ("error out"=w265:errorcluster, "index"=w267:i32, "String"=w269:string)  [unwired: 6 in]
        n118 = Unbundle By Name(w266) -> ("controls"=w257:T8)
        n119 = for {
          tunnel: w257 -> [w284] mode=indexing
          tunnel: [w278] -> w253
          stop <- w278 stop-if-true
          n120 = Unbundle By Name(w284) -> ("numero_misure_necessarie"=w283:u16, "numero_misure_effettuate"=w282:u32)
          n121 = Less Or Equal?(x=w283, y=w282) -> (x <= y?=w281:bool)
          n122 = Select(t=FALSE, s=w281, f=TRUE) -> (s? t:f=w278:bool)
        }
        n123 = Build Array(w255) -> (w254:refnum<vi>[])
        n124 = call "DisableControls.vi"("Visible"=w253, "Controls"=w254) -> ()  [unwired: 9 in, 1 out]
        n125 = Index Array(array=w257) -> (element=w260:T9)  [unwired: 1 in]
        n126 = Array Size(array=w257) -> (size(s)=→"Tot Misurazioni":i32)
        n127 = Unbundle By Name(w260) -> ("numero_misure_effettuate"=w258:u32, "numero_misure_necessarie"=w259:u16)
        n128 = Format Into String(format string="%d/%d", error in=w265, w258, w259) -> (resulting string=w261:string, error out=w264:errorcluster)  [unwired: 1 in]
        n129 = Bundle By Name(cluster=w273, "ByteGSAPIBase in"=w271, "Calibrations"=w266, "Misurazioni"=w269, "Misurazioni index"=w267, "Misurazioni n"=w261, "Misure effettuate"=w258) -> (w272:T7)
      }
      frame "CheckTotalMisurations" {
        n130 = Unbundle By Name(w291) -> ()  [unwired: 1 out]
        n131 = Unbundle By Name(w288) -> ("Calibrations"=w297:T3, "Cal Index"=w286:i32, "Misure effettuate"=w285:i32)
        n132 = Unbundle By Name(w297) -> ("controls"=w296:T8)
        n133 = Index Array(array=w296, index=w286) -> (element=w295:T9)
        n134 = Unbundle By Name(w295) -> ("numero_misure_necessarie"=w294:u16)
        n135 = Less Or Equal?(x=w294, y=w285) -> (x <= y?=w293:bool)
        n136 = case shown="True" w293 {
          tunnel: [CalibrationStates."StartCalibration" w302] -> w292
          tunnel: w290 -> [w299 w313]
          tunnel: [w299 w310] -> w289
          tunnel: w288 -> [w298 w315]
          tunnel: [w298 w309] -> w287
          tunnel: w286 -> [_ _]
          frame False {
          }
          frame True {
            n137 = Unbundle By Name(w315) -> ("Misure effettuate"=w317:i32, "Cal Index"=w306:i32, "Waveform Chart"=w312:refnum<vi>, "Calibrations"=w321:T3)
            n138 = Unbundle By Name(w321) -> ("controls"=w308:T8)
            n139 = Index Array(array=w308, index=w306) -> (element=w320:T9)
            n140 = Unbundle By Name(w320) -> ("numero_misure_necessarie"=w319:u16)
            n141 = property class="WFChart (strict)"(reference=w312, error in=w313, "History Data"=dbl[] []) -> (error out=w311:errorcluster)  [unwired: 1 out]
            n142 = Less Or Equal?(x=w319, y=w317) -> (x <= y?=w318:bool)
            n143 = case shown="True" w318 {
              tunnel: w306 -> [w328 w333]
              tunnel: [w328 w332] -> w326
              tunnel: w317 -> [w327 _]
              tunnel: [w327 w329] -> w316
              tunnel: w308 -> [_ w331]
              frame False {
              }
              frame True {
                n144 = Increment(x=w333) -> (x+1=w332:i32)
                n145 = Index Array(array=w331, index=w332) -> (element=w330:T9)
                n146 = Unbundle By Name(w330) -> ("numero_misure_effettuate"=w329:u32)
              }
            }
            n147 = Array Size(array=w308) -> (size(s)=w307:i32)
            n148 = Decrement(x=w307) -> (x-1=w301:i32)
            n149 = Less Or Equal?(x=w301, y=w306) -> (x <= y?=w305:bool)
            n150 = call "MisurazioniString.vi"("error in (no error)"=w311, "index"=w326, "Calibration data"=w321) -> ("error out"=w310:errorcluster, "index"=w324:i32, "String"=w325:string)  [unwired: 6 in]
            n151 = Bundle By Name(cluster=w315, "Misure effettuate"=w316, "Cal Index"=w326, "Misurazioni"=w325, "Misurazioni index"=w324, "Id Failed"=u32 0, "Failed?"=FALSE) -> (w309:T7)
            n152 = Select(t=CalibrationStates."AllowApprove", s=w305, f=CalibrationStates."CheckTotalMisurations") -> (s? t:f=w302:T2)
          }
        }
      }
      frame "StartCalibration" {
        n153 = Unbundle By Name(w347) -> ("Esito"=w346:refnum<vi>, "Avanti"=w334:refnum<vi>)
        n154 = Build Array(w334) -> (w336:refnum<vi>[])
        n155 = property class="Str"(reference=w346, error in=w343, "Text.BGColor"=u32 9678034 ("Text.Text Colors:BG Color")) -> (error out=w344:errorcluster)  [unwired: 1 out]
        n156 = Unbundle By Name(w359) -> ("Calibrations"=w363:T3, "New Val"=w356:dbl, "Cal Index"=w341:i32, "Misure effettuate"=w338:i32)  [unwired: 1 out]
        n157 = call "DisableControls.vi"("Visible"=FALSE, "Controls"=w336) -> ()  [unwired: 9 in, 1 out]
        n158 = Unbundle By Name(w363) -> ("controls"=w342:T8)
        n159 = call "FGVTimer.vi"("error in"=w344) -> ("error out"=w352:errorcluster, "Elapsed?"=w360:bool)  [unwired: 8 in, 1 out]
        n160 = Index Array(array=w342, index=w341) -> (element=w362:T9)
        n161 = Unbundle By Name(w362) -> ("riferimento_obiettivo"=w354:dbl)
        "Valore di riferimento" <- w354
        n162 = Index Array(array=w342, index=w341) -> (element=w340:T9)
        n163 = Unbundle By Name(w340) -> ("numero_misure_necessarie"=w339:u16)
        n164 = case shown="False" w360 {
          tunnel: w354 -> [w370 _]
          tunnel: [CalibrationStates."StartCalibration" CalibrationStates."ManageCalibration"] -> w357
          tunnel: [w364 w373] -> w355
          tunnel: w356 -> [_ w373]
          frame False {
            n165 = Quotient & Remainder(x=w370, y=10.0) -> (floor(x/y)=w369:dbl)  [unwired: 1 out]
            n166 = Add(x=w370, y=w369) -> (x+y=w368:dbl)
            n167 = Subtract(x=w370, y=w369) -> (x-y=w365:dbl)
            n168 = To Quad Integer(1:w368) -> (0:w367:i64)
            n169 = To Quad Integer(1:w365) -> (0:w366:i64)
            n170 = call-poly <vilib>:"Random Number (Range).vi"("lower bound (-100)"=w366, "upper bound (100)"=w367) -> ("number"=w364:i64)  [unwired: 9 in]
            "Waveform Chart" <- w364
          }
          frame True {
          }
        }
        "Valore misurato" <- w355
        n171 = Increment(x=w338) -> (x+1=w337:i32)
        n172 = Format Into String(format string="%d/%d", error in=w352, w337, w339) -> (resulting string=w350:string, error out=w351:errorcluster)  [unwired: 1 in]
        n173 = Bundle By Name(cluster=w359, "Next State"=w357, "New Val"=w355, "Misurazioni n"=w350, "Stato"="Calibrazione in corso", "Esito"="...") -> (w358:T7)
      }
      frame "ManageCalibration" {
        n174 = Unbundle By Name(w395) -> ("ByteGSAPIBase in"=w398:refnum<class "ByteGSAPIBase.lvclass">, "Calibrations.controls"=w401:T8, "New Val"=w397:dbl, "Id Failed"=w393:u32, "Failed?"=w390:bool, "Cal Index"=w380:i32, "Misure effettuate"=w378:i32)
        n175 = Unbundle By Name(w387) -> ("Repeat"=w376:refnum<vi>, "Avanti"=w377:refnum<vi>, "Esito"=w384:refnum<vi>)
        n176 = Index Array(array=w401, index=w380) -> (element=w400:T9)
        n177 = Unbundle By Name(w400) -> ("id"=w399:u16, "riferimento_obiettivo"=w396:dbl)
        n178 = disable-structure shown="Disabled" {
          disable-tunnel: w399 -> [w441 _]
          disable-tunnel: w398 -> [w440 w458]
          disable-tunnel: w397 -> [w439 w460]
          disable-tunnel: w396 -> [w438 w461]
          disable-tunnel: w381 -> [w437 w459]
          disable-tunnel: [w433 w459] -> w383
          disable-tunnel: w393 -> [w431 _]
          disable-tunnel: [w430 w458] -> w392
          disable-tunnel: [w429 _] -> w391
          disable-tunnel: w390 -> [w428 _]
          disable-tunnel: [w427 w456] -> w379
          frame Disabled {
            n179 = case shown="True" w428 {
              tunnel: w440 -> [w448 w455]
              tunnel: w438 -> [w447 _]
              tunnel: w439 -> [w446 w453]
              tunnel: w437 -> [w445 w454]
              tunnel: [w444 w451] -> w436
              tunnel: w441 -> [w442 w450]
              tunnel: [w443 w452] -> w435
              tunnel: [w442 w450] -> w434
              tunnel: w431 -> [_ w449]
              frame False {
                n180 = call-dynamic "AddMeasurement.vi"("measurement_group id"=w442, "error in (no error)"=w445, "misura_strumento"=w446, "misura_riferimento"=w447, "ByteGSAPIBase in"=w448) -> ("error out"=w444:errorcluster, "ByteGSAPIBase out"=w443:refnum<class "ByteGSAPIBase.lvclass">)  [unwired: 4 in, 1 out]
              }
              frame True {
                n181 = call-dynamic "EditMeasurement.vi"("error in (no error)"=w454, "instrument measure"=w453, "measurement id"=w449, "ByteGSAPIBase in"=w455) -> ("error out"=w451:errorcluster, "ByteGSAPIBase out"=w452:refnum<class "ByteGSAPIBase.lvclass">)  [unwired: 5 in, 1 out]
              }
            }
            n182 = call "MeasGroupResult.vi"("error in (no error)"=w436, "measurement_group_id"=w434, "ByteGSAPIBase in"=w435) -> ("error out"=w433:errorcluster, "measurements"=w432:cluster{"id":u32, "passed":bool}[], "ByteGSAPIBase out"=w430:refnum<class "ByteGSAPIBase.lvclass">)  [unwired: 5 in, 1 out]
            n183 = call "GetResult.vi"("measurements"=w432) -> ("passed"=w427:bool, "id"=w429:u32)  [unwired: 1 in]
          }
          frame Enabled {
            n184 = Equal?(x=w461, y=w460) -> (x = y?=w457:bool)
            n185 = Not(x=w457) -> (.not. x?=w456:bool)
          }
        }
        n186 = case shown="False" w379 {
          tunnel: ["Passato" ("Esito") "Fallito" ("Esito")] -> w385
          tunnel: w384 -> [w420 w424]
          tunnel: w383 -> [w418 w423]
          tunnel: [w417 w422] -> w382
          frame False {
            n187 = property class="Str"(reference=w420, error in=w418, "Text.BGColor"=u32 5558784 ("Text.Text Colors:BG Color")) -> (error out=w417:errorcluster)  [unwired: 1 out]
          }
          frame True {
            n188 = property class="Str"(reference=w424, error in=w423, "Text.BGColor"=u32 16737380 ("Text.Text Colors:BG Color")) -> (error out=w422:errorcluster)  [unwired: 1 out]
          }
        }
        n189 = case shown="True" w379 {
          tunnel: w378 -> [w409 w416]
          tunnel: [w408 w416] -> w375
          tunnel: w376 -> [w403 w411]
          tunnel: w377 -> [w402 w410]
          frame False {
            n190 = Build Array(w402) -> (w405:refnum<vi>[])
            n191 = Build Array(w403) -> (w407:refnum<vi>[])
            n192 = Increment(x=w409) -> (x+1=w408:i32)
            n193 = call "DisableControls.vi"("Visible"=FALSE, "Controls"=w407) -> ()  [unwired: 9 in, 1 out]
            n194 = call "DisableControls.vi"("Visible"=TRUE, "Controls"=w405) -> ()  [unwired: 9 in, 1 out]
          }
          frame True {
            n195 = Build Array(w411) -> (w415:refnum<vi>[])
            n196 = Build Array(w410) -> (w413:refnum<vi>[])
            n197 = call "DisableControls.vi"("Visible"=TRUE, "Controls"=w415) -> ()  [unwired: 9 in, 1 out]
            n198 = call "DisableControls.vi"("Visible"=FALSE, "Controls"=w413) -> ()  [unwired: 9 in, 1 out]
          }
        }
        n199 = Bundle By Name(cluster=w395, "ByteGSAPIBase in"=w392, "Id Failed"=w391, "Failed?"=w379, "Next State"=CalibrationStates."Idle", "Stato"="Risultato calibrazione", "Esito"=w385, "Misure effettuate"=w375) -> (w394:T7)
      }
      frame "AllowApprove" {
        n200 = Unbundle By Name(w471) -> ("Repeat"=w470:refnum<vi>, "Approvation"=w468:refnum<vi>, "Avanti"=w469:refnum<vi>)
        n201 = Unbundle By Name(w462) -> ("Calibrations.controls"=w463:T8, "Misure effettuate"=w467:i32, "Cal Index"=w466:i32)
        n202 = Array Size(array=w463) -> (size(s)=w478:i32)
        n203 = Decrement(x=w478) -> (x-1=w477:i32)
        n204 = Index Array(array=w463, index=w466) -> (element=w476:T9)
        n205 = Less Or Equal?(x=w477, y=w466) -> (x <= y?=w473:bool)
        n206 = Unbundle By Name(w476) -> ("numero_misure_necessarie"=w475:u16)
        n207 = Equal?(x=w467, y=w475) -> (x = y?=w474:bool)
        n208 = And(x=w474, y=w473) -> (x .and. y?=w472:bool)
        n209 = case shown="True" w472 {
          tunnel: w468 -> [_ w482]
          tunnel: w469 -> [_ w485]
          tunnel: w470 -> [_ w479]
          frame False {
          }
          frame True {
            n210 = Build Array(w482) -> (w481:refnum<vi>[])
            n211 = Build Array(w485, w479) -> (w484:refnum<vi>[])
            n212 = call "DisableControls.vi"("Visible"=TRUE, "Controls"=w481) -> ()  [unwired: 9 in, 1 out]
            n213 = call "DisableControls.vi"("Visible"=FALSE, "Controls"=w484) -> ()  [unwired: 9 in, 1 out]
          }
        }
      }
      frame "Approve" {
        n214 = Unbundle By Name(w492) -> ("Approvation"=w491:refnum<vi>)
        n215 = Build Array(w491) -> (w490:refnum<vi>[])
        n216 = call "DisableControls.vi"("Visible"=FALSE, "Controls"=w490) -> ()  [unwired: 9 in, 1 out]
        n217 = disable-structure shown="Disabled" {
          disable-tunnel: w496 -> [w497 w508]
          disable-tunnel: w495 -> [w500 w507]
          disable-tunnel: [w499 w508] -> w488
          disable-tunnel: [w498 w507] -> w493
          frame Disabled {
            n218 = in-place {
              in-place-border: w497 -> [w504]
              in-place-border: [w503] -> w498
              in-place-border: w500 -> [w501]
              n219 = in-place-cluster #2(w497) -> ("ByteGSAPIBase in"=w506:refnum<class "ByteGSAPIBase.lvclass">)
              n220 = Unbundle By Name(w504) -> ("Selected Slug"=w502:i32)
              n221 = call "RequestApproval.vi"("error in (no error)"=w501, "calibration_id"=w502, "ByteGSAPIBase in"=w506) -> ("error out"=w503:errorcluster, "ByteGSAPIBase out"=w505:refnum<class "ByteGSAPIBase.lvclass">)  [unwired: 6 in, 1 out]
              n222 = in-place-cluster #2("ByteGSAPIBase in"=w505) -> (w499:T7)
            }
          }
          frame Enabled {
          }
        }
        n223 = Bundle By Name(cluster=w488, "Stato"="Approvazione inviata") -> (w487:T7)
      }
    }
    n224 = Unbundle By Name(w37) -> ("Misurazioni"=→"Calibrazioni n.":string, "Misurazioni n"=→"Misurazione n.":string, "Stato"=→"Stato":string, "Esito"=→"Esito":string)
  }
